vi "5. 绘制：管道内的 光纤分布 图.vi"(0 "光纤：前段 颜色":u32(colorbox)=6927784, 1 "光纤：前段 填充?(F)":bool caption="光纤：前段 填充？(F)", 3 "光纤：后段 填充?(F) 2":bool caption="光纤：后段 填充？(F)", 5 "光纤：后段 颜色":u32(colorbox)=14780529, 7 "涂色分段：前段长度":i32=140, 9 "管道分布":picture, 11 "输入：放大":i32, 12 "光纤：后段 画笔":T1={"Width"=8, "Style"=enum."Solid"}, 13 "光纤分布":dbl[][](array[numeric]), 14 "光纤：前段 画笔":T1={"Width"=8, "Style"=enum."Solid"}) -> (4 "显示：管道+光纤分布":picture)   [LabVIEW 2018]
panel:
  in  "初始直线起点":cluster{"x":i16, "y":i16}[](array[cluster]) caption="直线结束点"
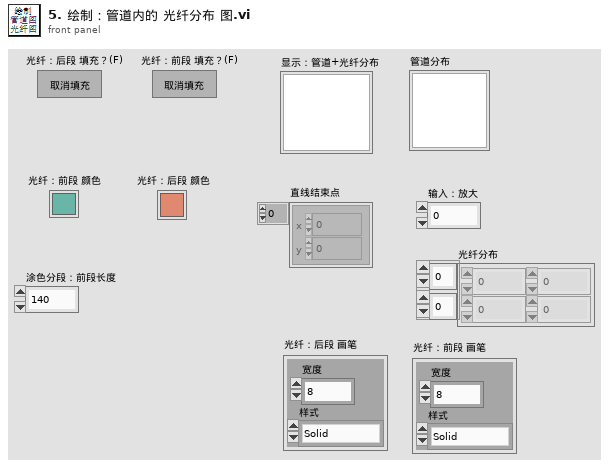
[diagram p1: front panel]
types:
  T1 = cluster{"Width":u16, "Style":enum32{"Solid", "Dash", "Dot", "DashDot", "DashDotDot"}}
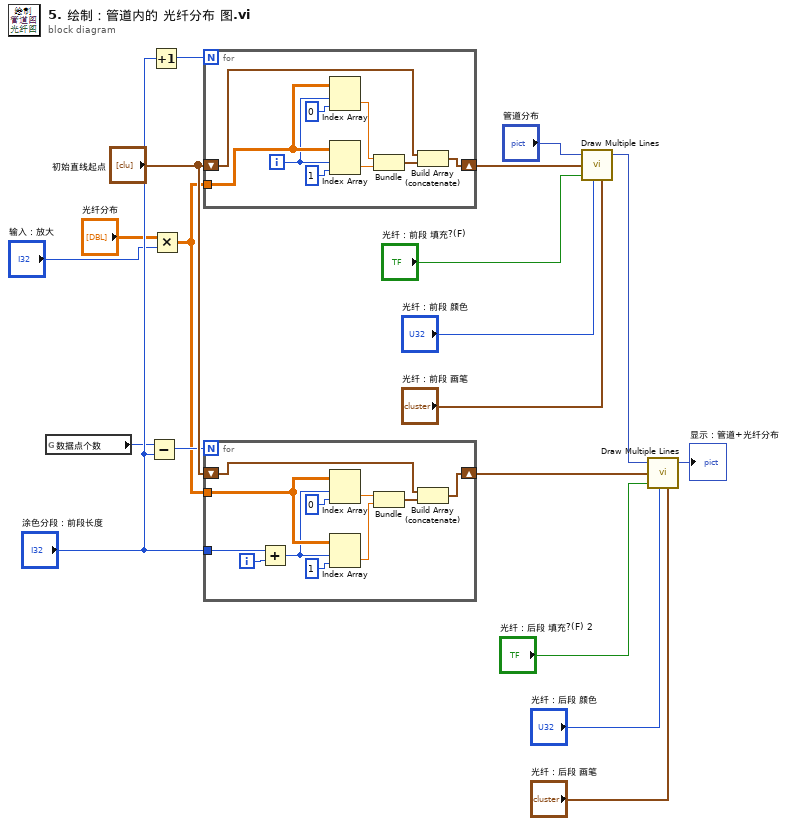
[diagram p0: block diagram]
diagram:
  n1 = global read "全局变量：数据点个数.vi" "数据点个数"() -> (w1:i32)
  n2 = Subtract(x=w1, y="涂色分段：前段长度") -> (x-y=w15:i32)
  n3 = Increment(x="涂色分段：前段长度") -> (x+1=w18:i32)
  n4 = Multiply(x="光纤分布", y="输入：放大") -> (x*y=w14:dbl[][])
  n5 = for {
    N: w18 -> [_]
    tunnel: w14 -> [w28]
    shift-right: [w23] -> w5
    shift-left: "初始直线起点" -> [w24]
    i -> [w27]
    n6 = Index Array(array=w28, index (row)=w27, index (col)=0) -> (element=w21:dbl)
    n7 = Index Array(array=w28, index (row)=w27, index (col)=1) -> (element=w22:dbl)
    n8 = Bundle(w21, w22) -> (w20:cluster{dbl, dbl})  [unwired: 1 in]
    n9 = Build Array (concatenate)(w24, w20) -> (w23:cluster{"x":dbl, "y":dbl}[])
  }
  n10 = for {
    N: w15 -> [_]
    tunnel: w14 -> [w39]
    shift-right: [w35] -> w16
    shift-left: "初始直线起点" -> [w36]
    tunnel: "涂色分段：前段长度" -> [w29]
    i -> [w30]
    n11 = Add(x=w29, y=w30) -> (x+y=w31:i32)
    n12 = Index Array(array=w39, index (row)=w31, index (col)=0) -> (element=w33:dbl)
    n13 = Index Array(array=w39, index (row)=w31, index (col)=1) -> (element=w34:dbl)
    n14 = Bundle(w33, w34) -> (w32:cluster{dbl, dbl})  [unwired: 1 in]
    n15 = Build Array (concatenate)(w36, w32) -> (w35:cluster{"x":dbl, "y":dbl}[])
  }
  n16 = call <vilib>:"Draw Multiple Lines.vi"("picture"="管道分布", "line endpoints"=w5, "fill?(F)"="光纤：前段 填充?(F)", "color(black)"="光纤：前段 颜色", "pen"="光纤：前段 画笔") -> ("new picture"=w13:picture)  [unwired: 4 in]
  n17 = call <vilib>:"Draw Multiple Lines.vi"("picture"=w13, "line endpoints"=w16, "fill?(F)"="光纤：后段 填充?(F) 2", "color(black)"="光纤：后段 颜色", "pen"="光纤：后段 画笔") -> ("new picture"=→"显示：管道+光纤分布":picture)  [unwired: 4 in]
